vi "Main_Fun_Obtain Queue.vi"(8 "Error in":errorcluster, 11 "Queue Name":string) -> (0 "Error Out":errorcluster, 3 "Message Queues":T1)   [LabVIEW 2015]
uses:
  Control_Main_Message Queues.ctl
  Control_Main_QData.ctl
  Control_Main_Queue Action.ctl
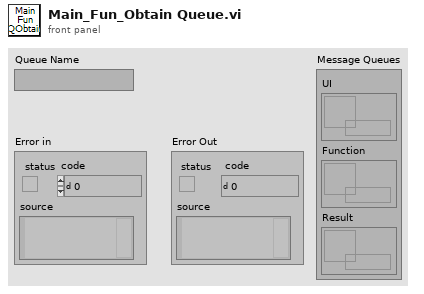
[diagram p1: front panel]
types:
  T1 = typedef "Control_Main_Message Queues.ctl" = cluster{"UI":refnum<queue>, "Function":refnum<queue>, "Result":refnum<queue>}
  T2 = typedef "Control_Main_QData.ctl" = cluster{"Queue Action":T3, "Queue Data":variant}
  T3 = typedef "Control_Main_Queue Action.ctl" = enum16{"動作-使用者登入", "動作-系統初始化", "動作-開始", "動作-系統管理選單", "動作-資料管理", "動作-登出/離開", "動作-關於本系統", "1.0 帳號管理", "    1.1 登入", "    1.2 確認狀態", "    1.3 更新介面", "    1.4 帳號管理", "    1.5 登出", "2.0 每日點檢", "10.0 系統", "    10.1 系統-關機", "    10.2 系統-等待", "    10.3 系統-回到作業系統"}
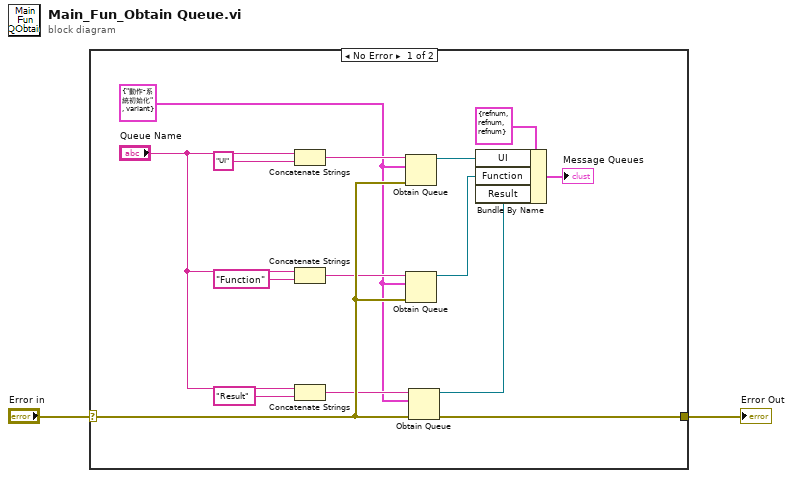
[diagram p0: block diagram]
diagram:
  n1 = case shown="No Error" "Error in" {
    selector: "Error in" -> [w17 w18]
    tunnel: [w5 w18] -> w1
    frame No Error {
      w6 = T2 {"Queue Action"=enum."動作-系統初始化", "Queue Data"=variant} ("Queue Data")
      n2 = Concatenate Strings("Queue Name", "UI" ("string")) -> (w16:string)
      n3 = Concatenate Strings("Queue Name", "Function" ("string")) -> (w15:string)
      n4 = Concatenate Strings("Queue Name", "Result" ("string")) -> (w14:string)
      n5 = Obtain Queue(name (unnamed)=w16, element data type=w6, error in (no error)=w17) -> (queue out=w9:refnum<queue>)  [unwired: 2 in, 2 out]
      n6 = Obtain Queue(name (unnamed)=w15, element data type=w6, error in (no error)=w17) -> (queue out=w8:refnum<queue>)  [unwired: 2 in, 2 out]
      n7 = Obtain Queue(name (unnamed)=w14, element data type=w6, error in (no error)=w17) -> (queue out=w7:refnum<queue>, error out=w5:errorcluster)  [unwired: 2 in, 1 out]
      n8 = Bundle By Name(cluster=T1 {"UI"=refnum, "Function"=refnum, "Result"=refnum} ("Message Queues"), "UI"=w9, "Function"=w8, "Result"=w7) -> (→"Message Queues":T1)
    }
    frame Error {
    }
  }
  "Error Out" <- w1
